vi "IB_RW_Project_Installer.vi"(7 "action":T1, 8 "error in (no error)":errorcluster, 9 "ProjectPath":path, 10 "Installer in":T2={"author"="", "productName"="", "buildSpecName"="", "hide"=FALSE, "requireLVDevSys"=FALSE, "autoIncrement"=FALSE, "includeError"=FALSE, "readmeID"="", "buildLocation"=path "", "mediaSize"=0, "language"=9, "productVersion"={"Major"=1, "Minor"=0, "Update"=0}, "defaultDir"="", "web service itemIDs"=[], "installerName"=""} {"productVersion"."Update" step=1; "productVersion"."Minor" step=1; "productVersion"."Major" step=1; "language" items=["English"=9, "German"=7, "French"=12, "Japanese"=17, "Korean"=18, "Chinese (Simplified)"=2052]}, 11 "Object In":T5) -> (0 "error out":errorcluster, 2 "Installer out":T2={"author"="", "productName"="", "buildSpecName"="", "hide"=FALSE, "requireLVDevSys"=FALSE, "autoIncrement"=FALSE, "includeError"=FALSE, "readmeID"="", "buildLocation"=path "", "mediaSize"=0, "language"=9, "productVersion"={"Major"=1, "Minor"=0, "Update"=0}, "defaultDir"="", "web service itemIDs"=[], "installerName"=""} {"productVersion"."Update" step=1; "productVersion"."Minor" step=1; "productVersion"."Major" step=1; "language" items=["English"=9, "German"=7, "French"=12, "Japanese"=17, "Korean"=18, "Chinese (Simplified)"=2052]}, 3 "Object Out":T5)   [LabVIEW 2020]
uses:
  <resource>/Framework/Providers/Builds/Installer/CDK_GLOBAL_STRINGS.vi
  <vilib>/AppBuilder/AB_Relative_Path_Type.ctl
  <resource>/Framework/Providers/API/ItemRef.ctl
  <vilib>/AppBuilder/IB_RW_Project/IB_RW_Project_Installer_Data.ctl
  <resource>/Framework/Providers/Builds/Installer/CDK_sTypeDef_Languages.ctl
  <resource>/Framework/Providers/Builds/Installer/CDK_sTypeDef_ProductVersion.ctl
  <vilib>/AppBuilder/IB_RW_Project/IB_RW_Project_PropBag_Action.ctl
panel:
  # "."
  # "."
  # "."
  # "."
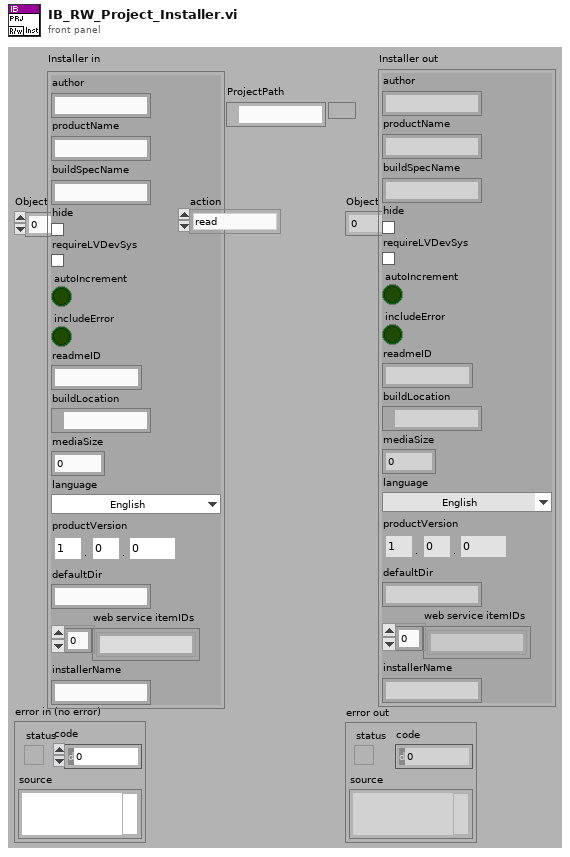
[diagram p1: front panel]
types:
  T1 = typedef "IB_RW_Project_PropBag_Action.ctl" = enum16{"read", "write", "clear", "readPrevious", "writePrevious", "clearPrevious"}
  T2 = typedef "IB_RW_Project_Installer_Data.ctl" = cluster{"author":string, "productName":string, "buildSpecName":string, "hide":bool, "requireLVDevSys":bool, "autoIncrement":bool, "includeError":bool, "readmeID":string, "buildLocation":path, "mediaSize":u16, "language":T3, "productVersion":T4, "defaultDir":string, "web service itemIDs":string[], "installerName":string}
  T3 = typedef "CDK_sTypeDef_Languages.ctl" = u16
  T4 = typedef "CDK_sTypeDef_ProductVersion.ctl" = cluster{"Major":u8, "Minor":u8, "Update":u16}
  T5 = typedef "ItemRef.ctl" = u64
  T6 = typedef "AB_Relative_Path_Type.ctl" = enum16{"<none>", "relativeToCommon", "relativeToAppDir", "relativeToProject"}
  T7 = typedef "IB_Relative_Path_Type.ctl" = enum16{"<none>", "relativeToCommon", "relativeToAppDir", "relativeToProject"}
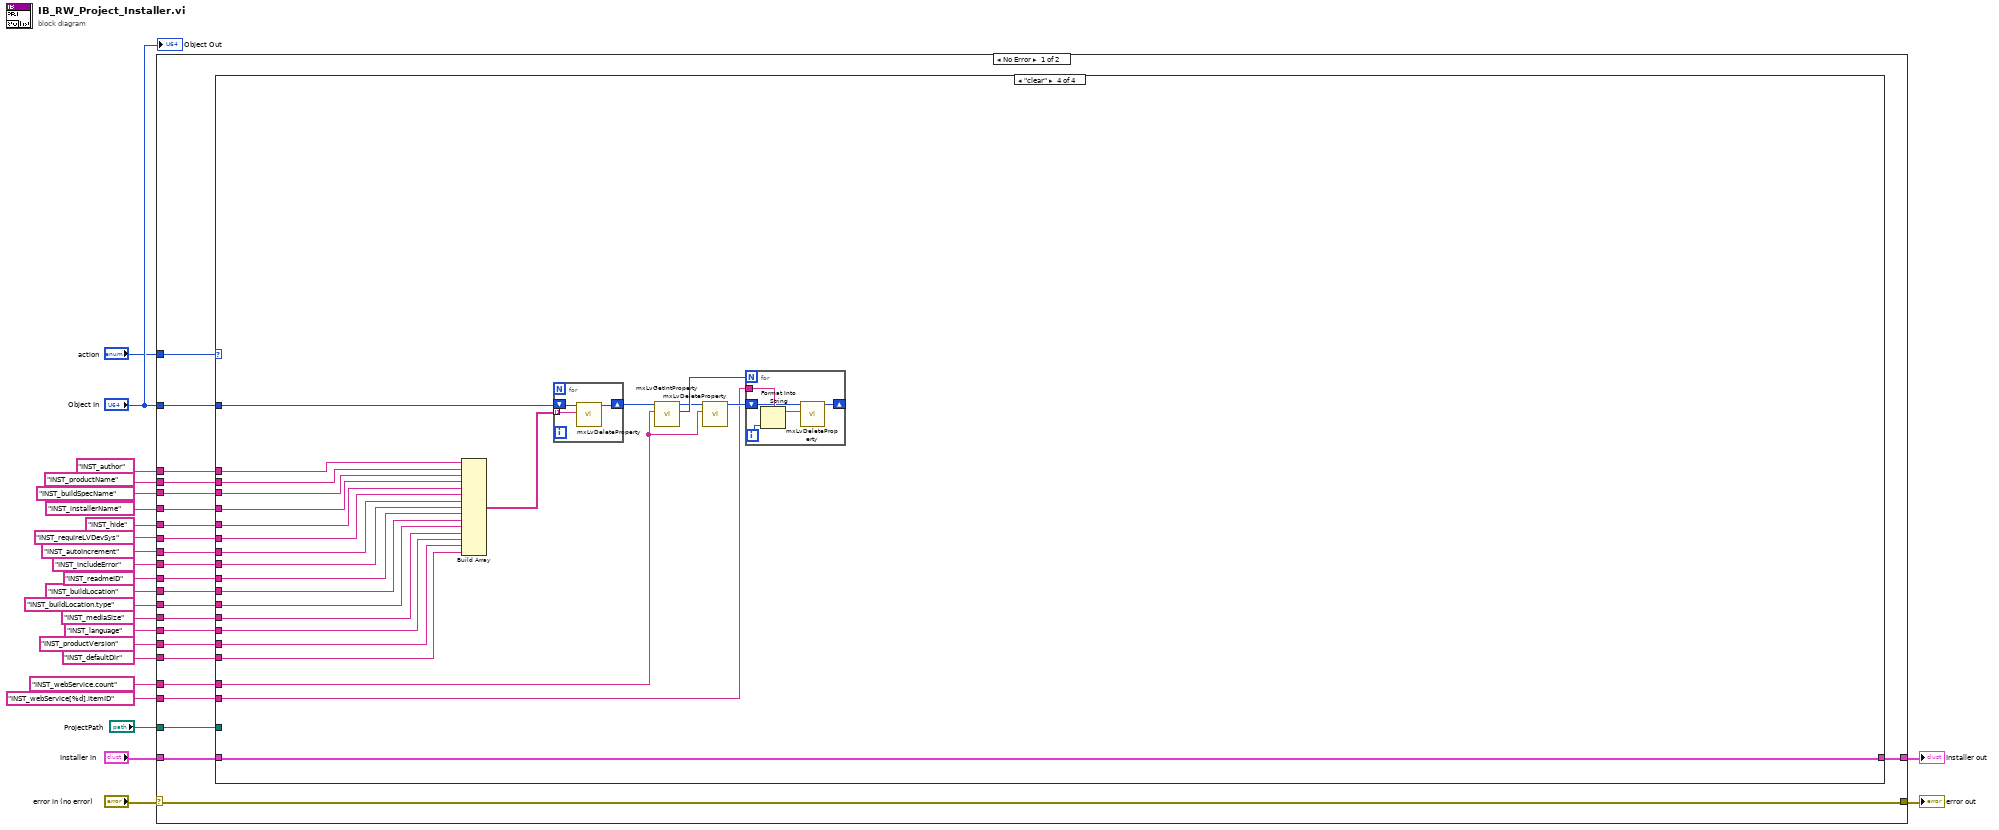
[diagram p0: block diagram]
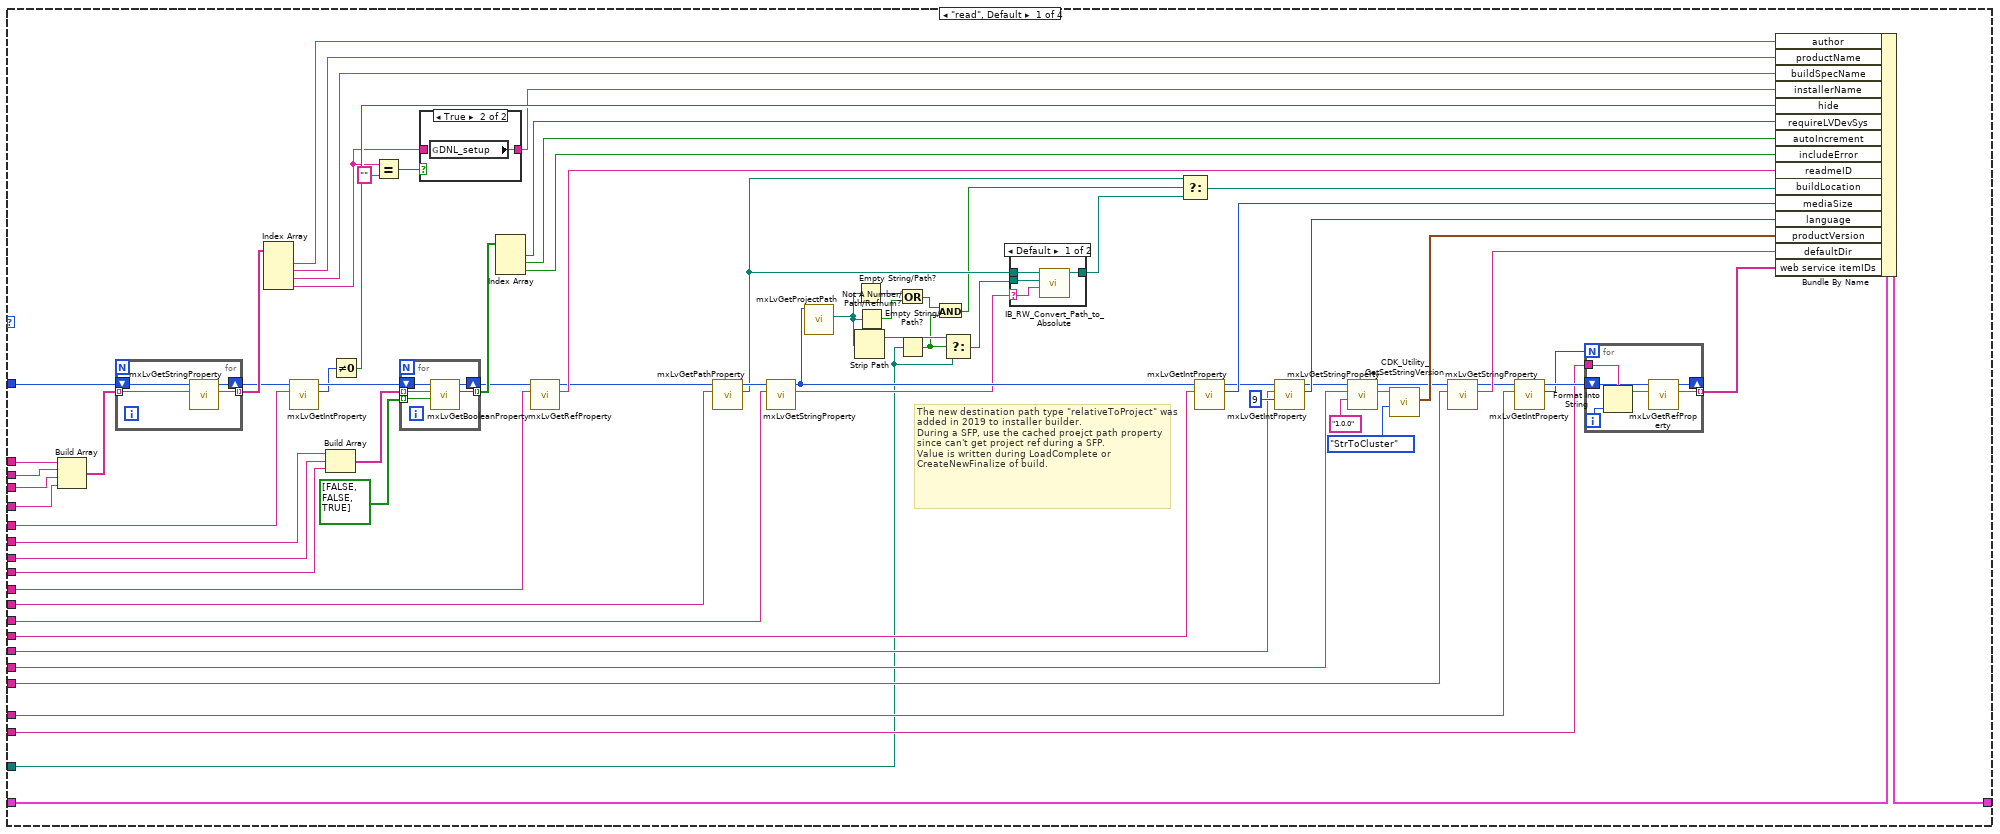
[diagram p2: hidden frame]
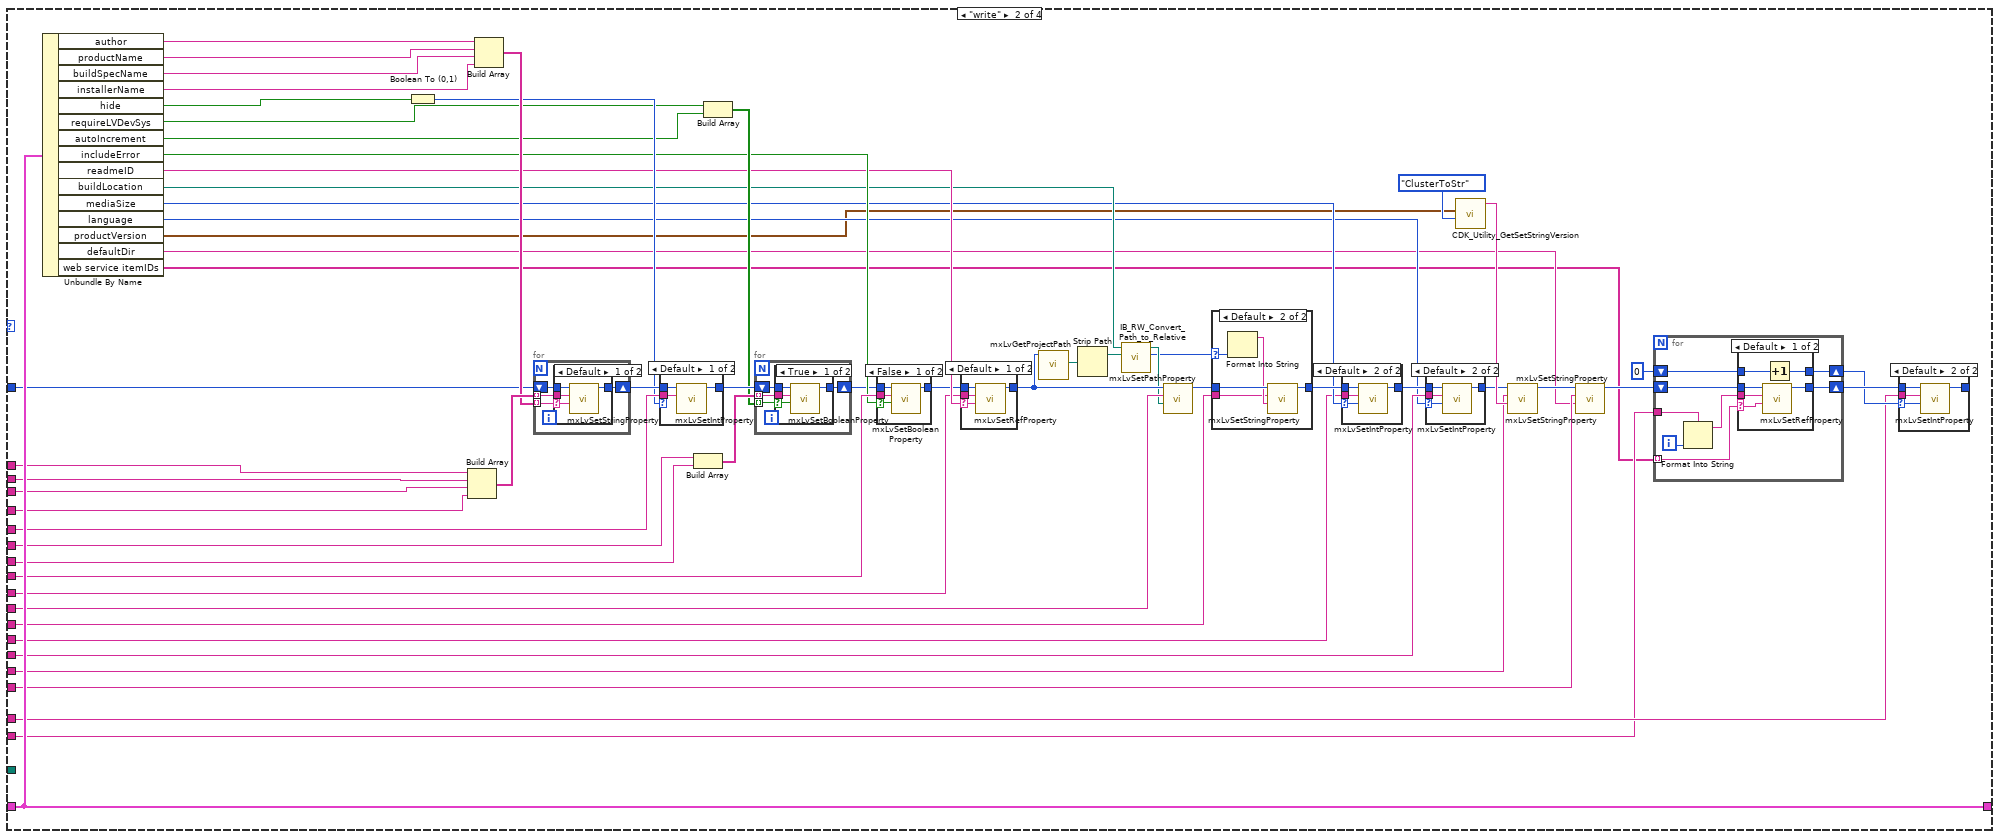
[diagram p5: hidden frame]
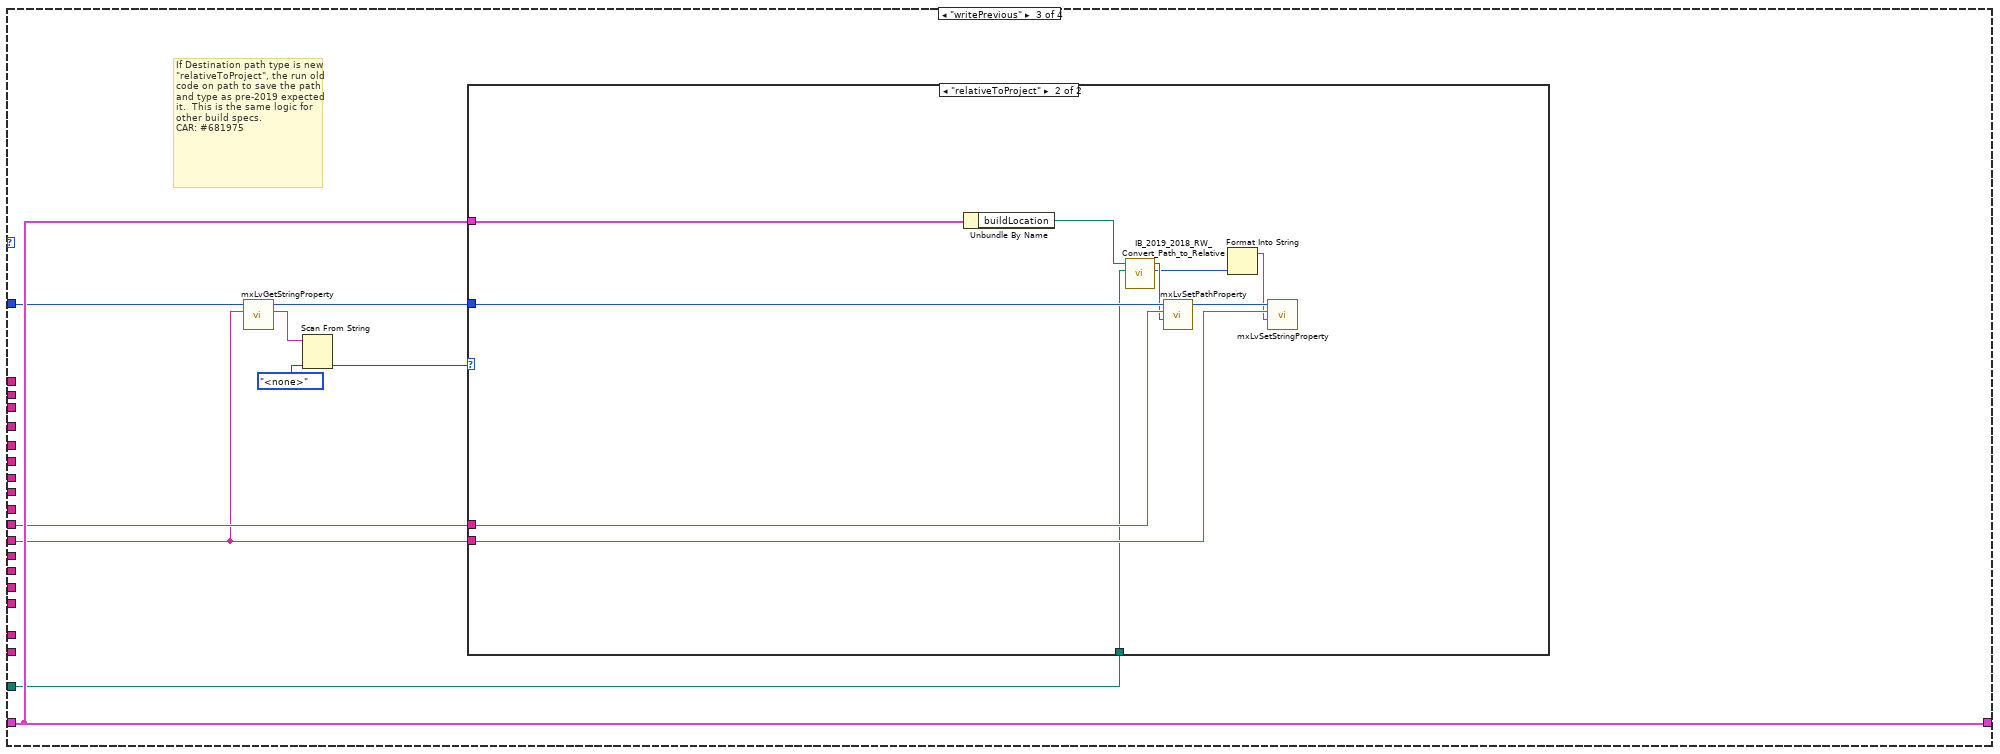
[diagram p16: hidden frame]
diagram:
  n1 = case shown="No Error" "error in (no error)" {
    selector: "error in (no error)" -> [w30 w321]
    tunnel: "Object In" -> [w29 _]
    tunnel: [w46 _] -> w22
    tunnel: "INST_author" ("Tag") -> [w44 _]
    tunnel: "INST_productName" ("Tag") -> [w43 _]
    tunnel: "INST_requireLVDevSys" ("Tag") -> [w40 _]
    tunnel: "INST_autoIncrement" ("Tag") -> [w39 _]
    tunnel: "INST_includeError" ("Tag") -> [w38 _]
    tunnel: "INST_readmeID" ("Tag") -> [w37 _]
    tunnel: "INST_buildLocation" ("Tag") -> [w36 _]
    tunnel: "INST_mediaSize" ("Tag") -> [w35 _]
    tunnel: "Installer in" -> [w47 _]
    tunnel: "action" -> [w45 _]
    tunnel: "INST_buildSpecName" ("Tag") -> [w42 _]
    tunnel: "INST_hide" ("Tag") -> [w41 _]
    tunnel: "INST_language" ("Tag") -> [w34 _]
    tunnel: "INST_buildLocation.type" ("Tag") -> [w33 _]
    tunnel: "INST_productVersion" ("Tag") -> [w32 _]
    tunnel: [w30 w321] -> w6
    tunnel: "INST_defaultDir" ("Tag") -> [w31 _]
    tunnel: "INST_webService.count" ("Tag") -> [w28 _]
    tunnel: "INST_webService[%d].itemID" ("Tag") -> [w27 _]
    tunnel: "INST_installerName" ("Tag") -> [w26 _]
    tunnel: "ProjectPath" -> [w25 _]
    frame No Error {
      n2 = case shown="\"clear\"" w45 {
        tunnel: [w119 w200 w278 w307] -> w46
        tunnel: w29 -> [w73 w151 w274 w312]
        tunnel: w47 -> [w118 w200 w278 w307]
        tunnel: w44 -> [w117 w199 _ w310]
        tunnel: w43 -> [w116 w198 _ w309]
        tunnel: w42 -> [w115 w197 _ w308]
        tunnel: w41 -> [w105 w189 _ w306]
        tunnel: w40 -> [w102 w184 _ w305]
        tunnel: w39 -> [w101 w183 _ w304]
        tunnel: w38 -> [w100 w182 _ w303]
        tunnel: w37 -> [w96 w177 _ w302]
        tunnel: w36 -> [w94 w174 w277 w301]
        tunnel: w34 -> [w88 w162 _ w300]
        tunnel: w35 -> [w93 w164 _ w299]
        tunnel: w33 -> [w79 w167 w272 w298]
        tunnel: w32 -> [w82 w156 _ w297]
        tunnel: w31 -> [w76 w153 _ w296]
        tunnel: w28 -> [w64 w146 _ w292]
        tunnel: w27 -> [w63 w145 _ w290]
        tunnel: w26 -> [w62 w142 _ w289]
        tunnel: w25 -> [w52 _ w270 _]
        frame "read", Default {
          # "The new destination path type \"relativeToProject\" was added in 2019 to installer builder.\nDuring a SFP, use the cached proejct path property since can't get project ref during a SFP.\nValue is written during LoadComplete or CreateNewFinalize of build."
          n3 = Build Array(w117, w116, w115, w62) -> (w114:string[])
          n4 = for {
            tunnel: [w141] -> w113 mode=indexing
            tunnel: w114 -> [w140] mode=indexing
            shift-right: [w138] -> w107
            shift-left: w73 -> [w139]
            n5 = call <resource>:"mxLvGetStringProperty.vi"("Tag"=w140, "Item"=w139) -> ("Value"=w141:string, "Item"=w138:T5)  [unwired: 1 in, 7 out]
          }
          n6 = Index Array(array=w113) -> (element #1=w110:string, element #2=w109:string, element #3=w108:string, element #4=w58:string)  [unwired: 4 in]
          n7 = call <resource>:"mxLvGetIntProperty.vi"("Tag"=w105, "Item"=w107) -> ("Value"=w104:i32, "Item"=w106:T5)  [unwired: 1 in, 7 out]
          n8 = Build Array(w102, w101, w100) -> (w112:string[])
          n9 = Not Equal To 0?(x=w104) -> (x != 0?=w103:bool)
          n10 = Equal?(x=w58, y="") -> (x = y?=w61:bool)
          n11 = for {
            shift-right: [w134] -> w78
            shift-left: w106 -> [w137]
            tunnel: w112 -> [w136] mode=indexing
            tunnel: [w135] -> w111 mode=indexing
            tunnel: bool[] [FALSE, FALSE, TRUE] -> [w133] mode=indexing
            n12 = call <resource>:"mxLvGetBooleanProperty.vi"("Default Value (F)"=w133, "Tag"=w136, "Item"=w137) -> ("Value"=w135:bool, "Item"=w134:T5)  [unwired: 1 in, 6 out]
          }
          n13 = case shown="True" w61 {
            tunnel: [w125 w126] -> w59
            tunnel: w58 -> [w125 _]
            frame False {
            }
            frame True {
              n14 = global read "CDK_GLOBAL_STRINGS.vi" "DNL_setup"() -> (w126:string)
            }
          }
          n15 = Index Array(array=w111) -> (element #1=w99:bool, element #2=w98:bool, element #3=w97:bool)  [unwired: 3 in]
          n16 = call <resource>:"mxLvGetRefProperty.vi"("Tag"=w96, "Item"=w78) -> ("Value"=w95:string, "Item"=w70:T5)  [unwired: 1 in, 7 out]
          n17 = call <resource>:"mxLvGetPathProperty.vi"("Tag"=w94, "Item"=w70) -> ("Path"=w56:path, "Item"=w81:T5)  [unwired: 2 in, 6 out]
          n18 = call <resource>:"mxLvGetStringProperty.vi"("Tag"=w79, "Item"=w81) -> ("Value"=w57:string, "Item"=w80:T5)  [unwired: 1 in, 7 out]
          n19 = call <resource>:"mxLvGetProjectPath.vi"("Item"=w80) -> ("Project Path"=w55:path)  [unwired: 1 in, 9 out]
          n20 = Strip Path(path=w55) -> (stripped path=w53:path)  [unwired: 1 out]
          n21 = Empty String/Path?(string/path=w55) -> (empty?=w71:bool)
          n22 = Not A Number/Path/Refnum?(number/path/refnum=w55) -> (NaN/Path/Refnum?=w72:bool)
          n23 = Or(x=w71, y=w72) -> (x .or. y?=w50:bool)
          n24 = Empty String/Path?(string/path=w52) -> (empty?=w49:bool)
          n25 = And(x=w50, y=w49) -> (x .and. y?=w48:bool)
          n26 = Select(t=w53, s=w49, f=w52) -> (s? t:f=w51:path)
          n27 = case shown="Default" w57 {
            selector: w57 -> [w123 _]
            tunnel: [w122 w124] -> w54
            tunnel: w56 -> [w121 w124]
            tunnel: w51 -> [w120 _]
            frame Default {
              n28 = call <vilib>:"IB_RW_Convert_Path_to_Absolute.vi"("relativeType"=w123, "commonPath"=w120, "relativePath"=w121) -> ("absolute path"=w122:path)  [unwired: 7 in, 1 out]
            }
            frame "" {
            }
          }
          n29 = Select(t=w56, s=w48, f=w54) -> (s? t:f=w69:path)
          n30 = call <resource>:"mxLvGetIntProperty.vi"("Tag"=w93, "Item"=w80) -> ("Value"=w92:i32, "Item"=w90:T5)  [unwired: 1 in, 7 out]
          n31 = call <resource>:"mxLvGetIntProperty.vi"("Default Value (0)"=9 ("Default (0)"), "Tag"=w88, "Item"=w90) -> ("Value"=w89:i32, "Item"=w86:T5)  [unwired: 1 in, 6 out]
          n32 = call <resource>:"mxLvGetStringProperty.vi"("Default Value (\"\")"="1.0.0", "Tag"=w82, "Item"=w86) -> ("Value"=w84:string, "Item"=w77:T5)  [unwired: 1 in, 6 out]
          n33 = call <resource>:"CDK_Utility_GetSetStringVersion.vi"("Action"=enum16{"ClusterToStr", "StrToCluster"}."StrToCluster", "VersionStringIn"=w84) -> ("ProductVersionOut"=w83:T4)  [unwired: 2 in, 7 out]
          n34 = call <resource>:"mxLvGetStringProperty.vi"("Tag"=w76, "Item"=w77) -> ("Value"=w75:string, "Item"=w66:T5)  [unwired: 1 in, 7 out]
          n35 = call <resource>:"mxLvGetIntProperty.vi"("Tag"=w64, "Item"=w66) -> ("Value"=w67:i32, "Item"=w68:T5)  [unwired: 7 in, 1 out]
          n36 = for {
            N: w67 -> [_]
            tunnel: w63 -> [w132]
            shift-right: [w129] -> _
            shift-left: w68 -> [w130]
            tunnel: [w128] -> w65 mode=indexing
            i -> [w131]
            n37 = Format Into String(format string=w132, w131) -> (resulting string=w127:string)  [unwired: 2 in, 1 out]
            n38 = call <resource>:"mxLvGetRefProperty.vi"("Tag"=w127, "Item"=w130) -> ("Value"=w128:string, "Item"=w129:T5)  [unwired: 7 in, 1 out]
          }
          n39 = Bundle By Name(cluster=w118, "author"=w110, "productName"=w109, "buildSpecName"=w108, "installerName"=w59, "hide"=w103, "requireLVDevSys"=w99, "autoIncrement"=w98, "includeError"=w97, "readmeID"=w95, "buildLocation"=w69, "mediaSize"=w92, "language"=w89, "productVersion"=w83, "defaultDir"=w75, "web service itemIDs"=w65) -> (w119:T2)
        }
        frame "write" {
          n40 = Unbundle By Name(w200) -> ("author"=w195:string, "productName"=w194:string, "buildSpecName"=w193:string, "installerName"=w143:string, "hide"=w188:bool, "requireLVDevSys"=w181:bool, "autoIncrement"=w180:bool, "includeError"=w179:bool, "readmeID"=w178:string, "buildLocation"=w171:path, "mediaSize"=w165:u16, "language"=w161:T3, "productVersion"=w159:T4, "defaultDir"=w152:string, "web service itemIDs"=w144:string[])
          n41 = Boolean To (0,1)(Boolean=w188) -> (0, 1=w187:i16)
          n42 = Build Array(w199, w198, w197, w142) -> (w196:string[])
          n43 = Build Array(w195, w194, w193, w143) -> (w192:string[])
          n44 = for {
            shift-right: [w264] -> w190
            shift-left: w151 -> [w263]
            tunnel: w196 -> [w262] mode=indexing
            tunnel: w192 -> [w261] mode=indexing
            n45 = case shown="Default" w261 {
              selector: w261 -> [w266 _]
              tunnel: w263 -> [w268 w269]
              tunnel: [w267 w269] -> w264
              tunnel: w262 -> [w265 _]
              frame Default {
                n46 = call <resource>:"mxLvSetStringProperty.vi"("Value (\"\")"=w266, "Tag"=w265, "Item"=w268) -> ("Item"=w267:T5)  [unwired: 2 in, 6 out]
              }
              frame "" {
              }
            }
          }
          n47 = case shown="Default" w187 {
            tunnel: w190 -> [w250 w251]
            tunnel: [w249 w251] -> w186
            tunnel: w189 -> [w248 _]
            frame Default {
              n48 = call <resource>:"mxLvSetIntProperty.vi"("Tag"=w248, "Item"=w250) -> ("Item"=w249:T5)  [unwired: 3 in, 6 out]
            }
            frame 0 {
            }
          }
          n49 = Build Array(w184, w183) -> (w191:string[])
          n50 = Build Array(w181, w180) -> (w185:bool[])
          n51 = for {
            shift-right: [w255] -> w176
            shift-left: w186 -> [w254]
            tunnel: w191 -> [w253] mode=indexing
            tunnel: w185 -> [w252] mode=indexing
            n52 = case shown="True" w252 {
              selector: w252 -> [w257 _]
              tunnel: w254 -> [w259 w260]
              tunnel: [w258 w260] -> w255
              tunnel: w253 -> [w256 _]
              frame True {
                n53 = call <resource>:"mxLvSetBooleanProperty.vi"("Value (F)"=w257, "Tag"=w256, "Item"=w259) -> ("Item"=w258:T5)  [unwired: 2 in, 6 out]
              }
              frame False {
              }
            }
          }
          n54 = case shown="False" w179 {
            selector: w179 -> [w244 _]
            tunnel: w176 -> [w246 w247]
            tunnel: w182 -> [w245 _]
            tunnel: [w243 w247] -> w155
            frame False {
              n55 = call <resource>:"mxLvSetBooleanProperty.vi"("Value (F)"=w244, "Tag"=w245, "Item"=w246) -> ("Item"=w243:T5)  [unwired: 2 in, 6 out]
            }
            frame True {
            }
          }
          n56 = case shown="Default" w178 {
            selector: w178 -> [w240 _]
            tunnel: w155 -> [w241 w242]
            tunnel: w177 -> [w239 _]
            tunnel: [w238 w242] -> w173
            frame Default {
              n57 = call <resource>:"mxLvSetRefProperty.vi"("Value (\"\")"=w240, "Tag"=w239, "Item"=w241) -> ("Item"=w238:T5)  [unwired: 2 in, 6 out]
            }
            frame "" {
            }
          }
          n58 = call <resource>:"mxLvGetProjectPath.vi"("Item"=w173) -> ("Project Path"=w175:path)  [unwired: 1 in, 9 out]
          n59 = Strip Path(path=w175) -> (stripped path=w172:path)  [unwired: 1 out]
          n60 = call <vilib>:"IB_RW_Convert_Path_to_Relative.vi"("commonPath"=w172, "absolutePath"=w171) -> ("relativeType"=w168:T6, "newPath"=w170:path)  [unwired: 7 in, 1 out]
          n61 = call <resource>:"mxLvSetPathProperty.vi"("Path"=w170, "Tag"=w174, "Item"=w173) -> ("Item"=w169:T5)  [unwired: 2 in, 6 out]
          n62 = case shown="Default" w168 {
            selector: w168 -> [_ w233]
            tunnel: [w232 w237] -> w166
            tunnel: w169 -> [w232 w236]
            tunnel: w167 -> [_ w234]
            frame "<none>" {
            }
            frame Default {
              n63 = Format Into String(w233) -> (resulting string=w235:string)  [unwired: 3 in, 1 out]
              n64 = call <resource>:"mxLvSetStringProperty.vi"("Value (\"\")"=w235, "Tag"=w234, "Item"=w236) -> ("Item"=w237:T5)  [unwired: 2 in, 6 out]
            }
          }
          n65 = case shown="Default" w165 {
            selector: w165 -> [_ w230]
            tunnel: w166 -> [w227 w231]
            tunnel: w164 -> [_ w229]
            tunnel: [w227 w228] -> w163
            frame 0 {
            }
            frame Default {
              n66 = call <resource>:"mxLvSetIntProperty.vi"("Value (0)"=w230, "Tag"=w229, "Item"=w231) -> ("Item"=w228:T5)  [unwired: 2 in, 6 out]
            }
          }
          n67 = case shown="Default" w161 {
            selector: w161 -> [_ w225]
            tunnel: w163 -> [w222 w226]
            tunnel: w162 -> [_ w224]
            tunnel: [w222 w223] -> w157
            frame 9 {
            }
            frame Default {
              n68 = call <resource>:"mxLvSetIntProperty.vi"("Value (0)"=w225, "Tag"=w224, "Item"=w226) -> ("Item"=w223:T5)  [unwired: 2 in, 6 out]
            }
          }
          n69 = call <resource>:"CDK_Utility_GetSetStringVersion.vi"("Action"=enum16{"ClusterToStr", "StrToCluster"}."ClusterToStr", "ProductVersionIn"=w159) -> ("VersionStringOut"=w158:string)  [unwired: 2 in, 7 out]
          n70 = call <resource>:"mxLvSetStringProperty.vi"("Value (\"\")"=w158, "Tag"=w156, "Item"=w157) -> ("Item"=w154:T5)  [unwired: 2 in, 6 out]
          n71 = call <resource>:"mxLvSetStringProperty.vi"("Value (\"\")"=w152, "Tag"=w153, "Item"=w154) -> ("Item"=w147:T5)  [unwired: 2 in, 6 out]
          n72 = for {
            tunnel: w145 -> [w213]
            tunnel: w144 -> [w211] mode=indexing
            shift-right: [w209] -> w150
            shift-left: w147 -> [w210]
            shift-right: [w206] -> w148
            shift-left: 0 -> [w207]
            i -> [w212]
            n73 = Format Into String(format string=w213, w212) -> (resulting string=w208:string)  [unwired: 2 in, 1 out]
            n74 = case shown="Default" w211 {
              selector: w211 -> [w214 _]
              tunnel: w210 -> [w217 w221]
              tunnel: w208 -> [w215 _]
              tunnel: [w216 w221] -> w209
              tunnel: w207 -> [w219 w220]
              tunnel: [w218 w220] -> w206
              frame Default {
                n75 = call <resource>:"mxLvSetRefProperty.vi"("Value (\"\")"=w214, "Tag"=w215, "Item"=w217) -> ("Item"=w216:T5)  [unwired: 7 in, 1 out]
                n76 = Increment(x=w219) -> (x+1=w218:i32)
              }
              frame "" {
              }
            }
          }
          n77 = case shown="Default" w148 {
            selector: w148 -> [_ w203]
            tunnel: w150 -> [w201 w205]
            tunnel: [w201 w204] -> _
            tunnel: w146 -> [_ w202]
            frame 0 {
            }
            frame Default {
              n78 = call <resource>:"mxLvSetIntProperty.vi"("Value (0)"=w203, "Tag"=w202, "Item"=w205) -> ("Item"=w204:T5)  [unwired: 7 in, 1 out]
            }
          }
        }
        frame "writePrevious" {
          # "If Destination path type is new \"relativeToProject\", the run old code on path to save the path and type as pre-2019 expected it.  This is the same logic for other build specs.\nCAR: #681975"
          n79 = call <resource>:"mxLvGetStringProperty.vi"("Tag"=w272, "Item"=w274) -> ("Value"=w276:string, "Item"=w273:T5)  [unwired: 1 in, 7 out]
          n80 = Scan From String(input string=w276, default 1=AB_Relative_Path_Type."<none>" ("relativeType")) -> (output 1=w271:T6)  [unwired: 3 in, 3 out]
          n81 = case shown="\"relativeToProject\"" w271 {
            tunnel: w278 -> [_ w288]
            tunnel: w277 -> [_ w287]
            tunnel: w273 -> [_ w285]
            tunnel: w272 -> [_ w284]
            tunnel: w270 -> [_ w279]
            frame "<none>", Default {
            }
            frame "relativeToProject" {
              n82 = Unbundle By Name(w288) -> ("buildLocation"=w282:path)
              n83 = call <vilib>:"IB_2019_2018_RW_Convert_Path_to_Relative.vi"("commonPath"=w279, "absolutePath"=w282) -> ("relativeType"=w280:T7, "newPath"=w281:path)  [unwired: 7 in, 1 out]
              n84 = call <resource>:"mxLvSetPathProperty.vi"("Path"=w281, "Tag"=w287, "Item"=w285) -> ("Item"=w286:T5)  [unwired: 2 in, 6 out]
              n85 = Format Into String(w280) -> (resulting string=w283:string)  [unwired: 3 in, 1 out]
              n86 = call <resource>:"mxLvSetStringProperty.vi"("Value (\"\")"=w283, "Tag"=w284, "Item"=w286) -> ()  [unwired: 2 in, 7 out]
            }
          }
        }
        frame "clear" {
          n87 = Build Array(w310, w309, w308, w289, w306, w305, w304, w303, w302, w301, w298, w299, w300, w297, w296) -> (w311:string[])
          n88 = for {
            tunnel: w311 -> [w319] mode=indexing
            shift-right: [w318] -> w291
            shift-left: w312 -> [w320]
            n89 = call <resource>:"mxLvDeleteProperty.vi"("Tag"=w319, "Item"=w320) -> ("Item"=w318:T5)  [unwired: 1 in, 8 out]
          }
          n90 = call <resource>:"mxLvGetIntProperty.vi"("Tag"=w292, "Item"=w291) -> ("Value"=w295:i32, "Item"=w294:T5)  [unwired: 7 in, 1 out]
          n91 = call <resource>:"mxLvDeleteProperty.vi"("Tag"=w292, "Item"=w294) -> ("Item"=w293:T5)  [unwired: 1 in, 8 out]
          n92 = for {
            N: w295 -> [_]
            tunnel: w290 -> [w317]
            shift-right: [w313] -> _
            shift-left: w293 -> [w315]
            i -> [w316]
            n93 = Format Into String(format string=w317, w316) -> (resulting string=w314:string)  [unwired: 2 in, 1 out]
            n94 = call <resource>:"mxLvDeleteProperty.vi"("Tag"=w314, "Item"=w315) -> ("Item"=w313:T5)  [unwired: 1 in, 8 out]
          }
        }
      }
    }
    frame Error {
    }
  }
  "error out" <- w6
  "Installer out" <- w22
  "Object Out" <- "Object In"
